vi "BRig_RT__Case_Exp__State_SelectPre.vi"(0 "input_dataCurrent":u16[](array[numeric]), 1 "input_SelectWrong":bool, 2 "input_SelectReward":bool, 5 "input_dataExp":u16[](array[numeric]), 7 "input_LickL":bool, 9 "input_LickR":bool, 11 "input_arrTrig":bool[](array[boolean])) -> (3 "output_state":T1, 4 "output_dataCurrent":u16[](array[numeric]), 8 "output_l1_laserEvent":bool, 10 "output_l1_laserOn":bool, 13 "output_l2_laserOn":bool, 14 "output_l2_laserEvent":bool)   [LabVIEW 2014]
uses:
  myRIO_BRig_RT__Case_Exp_stateList.ctl
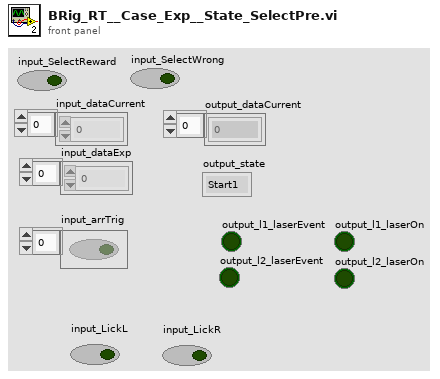
[diagram p1: front panel]
types:
  T1 = typedef "myRIO_BRig_RT__Case_Exp_stateList.ctl" = enum16{"Start1", "Start2", "Start3", "saveSettings1", "saveSettings2", "saveSettings3", "saveSettings4", "saveSettings_LC_ENL_l1", "saveSettings_LC_ENL_l2", "saveSettings_LC_Cue_l1", "saveSettings_LC_Cue_l2", "saveSettings6_LC_l1_Other", "SaveSettings6_LC_l2_Other", "setSettings_Audio", "setSettings_Laser", "initBlock_pre", "initBlock", "initBlock2", "initBlock_post", "initTrial_pre", "initTrial", "initTrial2", "initTrial3", "initTrial4", "initTrial_LC_ENL1", "initTrial_LC_Cue1", "initTrial_LC_Cue1_2", "initTrial_LC_Sel", "initTrial_post", "ENL1_pre", "ENL1", "ENL1_post", "ENL1Penalty_pre", "ENL1Penalty", "ENL2_pre", "ENL2", "ENL2Penalty_pre", "ENL2Penalty", "Cue1_pre", "Cue1", "Cue1_post", "Cue1Penalty_pre", "Cue1Penalty", "Cue2_pre", "Cue2", "Cue2Penalty_pre", "Cue2Penalty", "Selection_pre", "Selection", "Select_post", "SelectReward_pre", "SelectReward", "SelectRewardPost_pre", "SelectRewardPost", "SelectWrong_pre", "SelectWrong", "SelectWrong_post", "SelectTimeout_pre", "SelectTimeout", "SelectTimeout_post", "endTrial_pre", "endTrial1", "endTrial2", "endTrial3", "endTrial_post", "endBlock_pre", "endBlock", "endBlock_post", "endExp", "commConnect", "commUpload_pre", "commUpload_dataBlock", "commUpload_dataCurrent", "commUpload_dataExp", "commUpload_dataLC", "commUpload_dataTrial", "commUpload_post", "saveData_pre", "saveData_dataBlock", "saveData_dataCurrent", "saveData_dataExp", "saveData_dataLC", "saveData_dataTrial", "saveData_post", "empty_endBlock1", "empty_endBlock2", "empty_endTrial1", "empty_endTrial2", "empty_endTrial3", "empty_endTrial4", "empty_endTrial5", "dummyState", "dummyState_endBlock", "FreeReward_pre", "FreeReward", "FreeRewardPost_pre", "FreeRewardPost"}
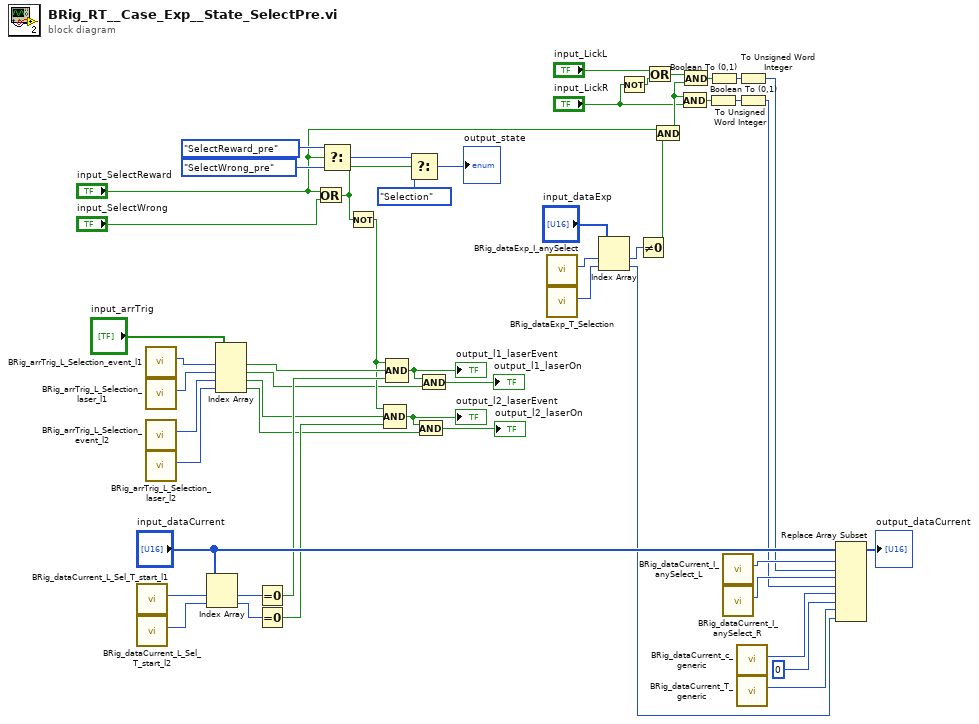
[diagram p0: block diagram]
diagram:
  n1 = call "BRig_dataCurrent_L_Sel_T_start_l1.vi"() -> ("output_L_Sel_T_start_l1"=w34:i32)  [unwired: 11 in]
  n2 = call "BRig_dataCurrent_L_Sel_T_start_l2.vi"() -> ("output_L_Sel_T_start_l2"=w35:i32)  [unwired: 11 in]
  n3 = call "BRig_arrTrig_L_Selection_event_l1.vi"() -> ("output_L_Sel_event_l1"=w11:i32)  [unwired: 11 in]
  n4 = call "BRig_arrTrig_L_Selection_laser_l1.vi"() -> ("output_L_Sel_laserTrig_l1"=w10:i32)  [unwired: 11 in]
  n5 = call "BRig_arrTrig_L_Selection_event_l2.vi"() -> ("output_L_Sel_event_l2"=w9:i32)  [unwired: 11 in]
  n6 = call "BRig_arrTrig_L_Selection_laser_l2.vi"() -> ("output_L_Sel_laserTrig_l2"=w8:i32)  [unwired: 11 in]
  n7 = Index Array(array="input_dataCurrent", index #1=w34, index #2=w35) -> (element #1=w48:u16, element #2=w47:u16)
  n8 = Index Array(array="input_arrTrig", index #1=w11, index #2=w10, index #3=w9, index #4=w8) -> (element #1=w41:bool, element #2=w4:bool, element #3=w42:bool, element #4=w6:bool)
  n9 = Equal To 0?(x=w48) -> (x = 0?=w46:bool)
  n10 = Equal To 0?(x=w47) -> (x = 0?=w45:bool)
  n11 = Or(x="input_SelectReward", y="input_SelectWrong") -> (x .or. y?=w33:bool)
  n12 = Select(t=myRIO_BRig_RT__Case_Exp_stateList."SelectReward_pre" ("Enum"), s="input_SelectReward", f=myRIO_BRig_RT__Case_Exp_stateList."SelectWrong_pre" ("Enum")) -> (s? t:f=w40:T1)
  n13 = Not(x=w33) -> (.not. x?=w32:bool)
  n14 = Compound Arithmetic op=AND(w32, w42, w45) -> (w7:bool)
  "output_l2_laserEvent" <- w7
  n15 = Compound Arithmetic op=AND(w32, w41, w46) -> (w5:bool)
  "output_l1_laserEvent" <- w5
  n16 = Select(t=w40, s=w33, f=myRIO_BRig_RT__Case_Exp_stateList."Selection" ("Enum")) -> (s? t:f=→"output_state":T1)
  n17 = And(x=w7, y=w6) -> (x .and. y?=→"output_l2_laserOn":bool)
  n18 = And(x=w5, y=w4) -> (x .and. y?=→"output_l1_laserOn":bool)
  n19 = call "BRig_dataExp_I_anySelect.vi"() -> ("output_I_anySelect"=w28:i32)  [unwired: 11 in]
  n20 = call "BRig_dataExp_T_Selection.vi"() -> ("output_T_Selection"=w29:i32)  [unwired: 11 in]
  n21 = Index Array(array="input_dataExp", index #1=w28, index #2=w29) -> (element #1=w27:u16, element #2=w1:u16)
  n22 = Not(x="input_LickR") -> (.not. x?=w13:bool)
  n23 = Not Equal To 0?(x=w27) -> (x != 0?=w26:bool)
  n24 = Or(x="input_LickL", y=w13) -> (x .or. y?=w12:bool)
  n25 = And(x="input_SelectReward", y=w26) -> (x .and. y?=w22:bool)
  n26 = And(x=w22, y="input_LickR") -> (x .and. y?=w20:bool)
  n27 = And(x=w12, y=w22) -> (x .and. y?=w21:bool)
  n28 = Boolean To (0,1)(Boolean=w20) -> (0, 1=w18:i16)
  n29 = Boolean To (0,1)(Boolean=w21) -> (0, 1=w19:i16)
  n30 = call "BRig_dataCurrent_I_anySelect_L.vi"() -> ("output_IanySelect_L"=w24:i32)  [unwired: 11 in]
  n31 = call "BRig_dataCurrent_I_anySelect_R.vi"() -> ("output_IanySelect_R"=w23:i32)  [unwired: 11 in]
  n32 = call "BRig_dataCurrent_c_generic.vi"() -> ("output_count_generic"=w51:i32)  [unwired: 11 in]
  n33 = call "BRig_dataCurrent_T_generic.vi"() -> ("output_T_generic"=w50:i32)  [unwired: 11 in]
  n34 = To Unsigned Word Integer(number=w19) -> (unsigned 16bit integer=w16:u16)
  n35 = To Unsigned Word Integer(number=w18) -> (unsigned 16bit integer=w17:u16)
  n36 = Replace Array Subset(array="input_dataCurrent", new element #1=w16, index #1=w24, new element #2=w17, index #2=w23, new element #3=u16 0 ("new element/subarray"), index #3=w51, new element #4=w1, index #4=w50) -> (→"output_dataCurrent":u16[])
